vi "Main.vi"() -> ()   [LabVIEW 2019, in "GameEngine.lvlib"]
uses:
  GameEngine.lvlib
  Sprite/SpriteData.ctl
  VGA/data.ctl
  <vilib>/Platform/TimedLoop/XDataNode/timing_clust.ctl
  <vilib>/Platform/TimedLoop/XDataNode/nitl_modes.ctl
  <vilib>/Platform/TimedLoop/XDataNode/wakeup.ctl
  <vilib>/rvi/Emulation/niFpgaGetClockAttributes.vi
  <vilib>/rvi/Emulation/niFpgaSctlEmulationGetInTimedLoop.vi
  <vilib>/rvi/Emulation/niFpgaEmulationReportErrorSimple.vi
  <vilib>/rvi/interface/RandomDataEmulation/niFpgaRandomDataHandleErrors.vi
  <vilib>/rvi/Emulation/niFpgaProcessEmulError.vi
  <vilib>/rvi/Emulation/niFpgaCriticalErrorInLSC.vi
  <vilib>/rvi/eio/common/nirviEmuTemplateMethod_errors.vi
  <vilib>/rvi/Memory/Memory_Emulation/nirvimemoryFastEmulation.vi
  <vilib>/rvi/Memory/Memory_Emulation/nirvimemoryEmulation.vi
  <vilib>/rvi/Emulation/niFpgaEmulationIsFPGAContextNoSignature.vi
  <vilib>/rvi/DataTransferAndStorage/Container/Common/niFpgaContainerGetUniqueNameForEmu.vi
  <vilib>/rvi/errors/nirviReportUnexpectedCaseInternalError (U32).vi
  <vilib>/rvi/DataTransferAndStorage/Container/Common/niFpgaContainerExecOnDevCompGetState.vi
  <vilib>/rvi/Memory/Memory_Emulation/niFpgaMemoryEmulationCacheClearOnFirstRun.vi
  <vilib>/rvi/Memory/Memory_Emulation/nirvimemoryEmulationManagerCache_MakeExclusive.vi
  <vilib>/rvi/Memory/Memory_Emulation/niFpgaMemoryEmulationValidateCache.vi
  <vilib>/rvi/Memory/Memory_Emulation/nirvimemoryEmulationManagerCache_InsertValue.vi
  <vilib>/Utility/error.llb/Clear Errors.vi
  <vilib>/rvi/Memory/Memory_Emulation/nirvimemoryEmulationManagerCache_ReleaseExclusive.vi
  <vilib>/rvi/Memory/Memory_Emulation/nirvimemoryEmulationManagerCache_GetValue.vi
  <vilib>/rvi/Memory/Memory_Emulation/nirvimemoryEmulationManagerCache_SetValue.vi
  <vilib>/rvi/Emulation/niFpgaSctlEmulationResourceMgr.vi
  <vilib>/rvi/DataTransferAndStorage/Container/XNode/niFpgaContainer.xnode
  <vilib>/rvi/interface/RandomDataEmulation/nirviRandomDataFpgaReadWriteTemplate.vi
  <vilib>/eio/EIONode/EIONode.xnode
  <vilib>/platform/TimedLoop/XDataNode/XDataNode.xnode
  <vilib>/rvi/Memory/Memory_Emulation/niFpgaMemoryEmulationRefIn.vi
  <vilib>/Platform/TimedLoop/XDataNode/XDNodeRunTimeDep.lvlib
  Shared/Shared.lvlib
  Sprite/Sprite.lvlib
  VGA/VGA.lvlib
panel:
  in  "y_Shift":i16
  in  "x_Shift":i16
  out "SoundBufferTimeout":bool
  out "SoundBufferFlushing":bool
  in  "SoundBuffer_Flush":bool
  in  "Spritebuffer_ResetAddress":bool
  in  "FadeColor":fxp<+,3,3>
  in  "FadeRate":u32=308000
  in  "ColorShift":fxp<+,3,3>
  in  "Tilebuffer_ResetAddress":bool
  in  "Sprites":T1[](array[typedef])=[{"Pos_X"=0, "Pos_Y"=0, "Width"=0, "Height"=0, "BufferIndex"=0, "TransparencyColor"=0.0}, {"Pos_X"=0, "Pos_Y"=0, "Width"=0, "Height"=0, "BufferIndex"=0, "TransparencyColor"=0.0}, {"Pos_X"=0, "Pos_Y"=0, "Width"=0, "Height"=0, "BufferIndex"=0, "TransparencyColor"=0.0}]
  out "right_2":bool
  out "right_1":bool
  out "right_down":bool
  out "right_up":bool
  out "right_right":bool
  out "right_left":bool
  out "SystemButton":bool
  out "left_2":bool
  out "left_1":bool
  out "left_down":bool
  out "left_up":bool
  out "left_right":bool
  out "left_left":bool
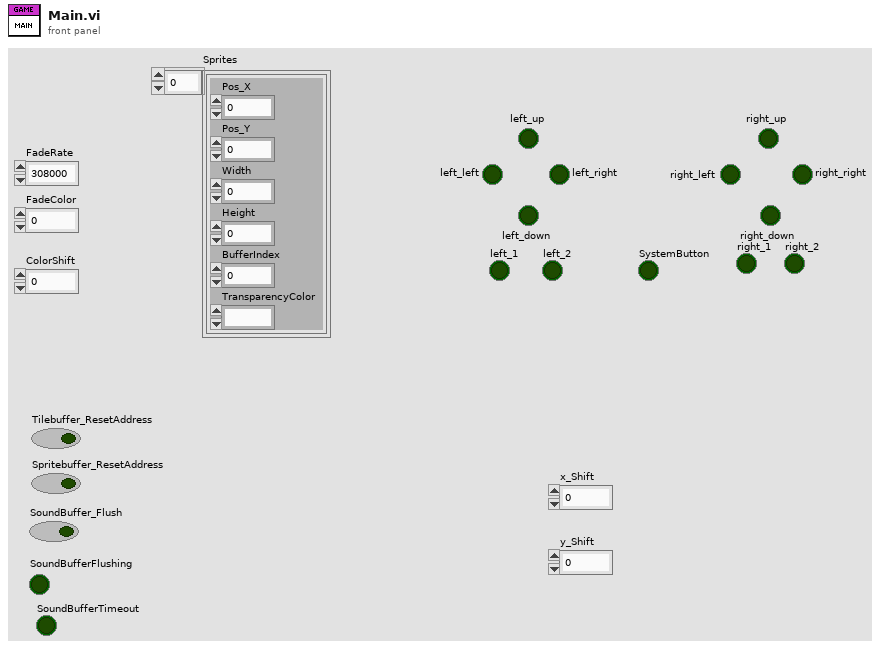
[diagram p1: front panel]
types:
  T1 = typedef "Sprite.lvlib/SpriteData.ctl" = cluster{"Pos_X":i16, "Pos_Y":i16, "Width":i16, "Height":i16, "BufferIndex":i16, "TransparencyColor":fxp<+,3,3>}
  T2 = typedef "VGA.lvlib/data.ctl" = cluster{"x_frontporch":u8, "x_syncpulse":u8, "x_backporch":u8, "y_frontporch":u8, "y_syncpulse":u8, "y_backporch":u8, "DrawPixel?":bool, "x_tickcount":u16, "y_tickcount":u16, "x_Index":i16, "y_Index":i16, "x_shift":i16}
  T3 = typedef "XDNodeRunTimeDep.lvlib/timing_clust.ctl" = cluster{"Expected End [f-1]":u64, "Actual End [f-1]":u64, "Finished Late? [f-1]":bool, "Expected End [i-1]":u64, "Actual End [i-1]":u64, "Finished Late? [i-1]":bool, "Expected Start [i]":u64, "Actual Start [i]":u64, "Expected Start [f]":u64, "Actual Start [f]":u64, "Source Name":string, "Structure Name":string, "Period":i64, "Deadline":i64, "Offset":i64, "Start":i64, "Priority":i32, "Timeout":i32, "Mode":T4, "Wakeup Reason":T5, "Error":errorcluster, "Source Type":string, "Secondary Source Type":string, "Global End Time":u64, "Global Start Time":u64, "Frame Duration":u64, "Iteration Duration":u64, "Assigned CPU":i32, "I/O Scan Engine Mode":u32}
  T4 = typedef "XDNodeRunTimeDep.lvlib/nitl_modes.ctl" = enum32{"No Change", "Process missed periods, maintain original phase", "Discard missed periods, maintain original phase", "Process missed periods, ignore original phase", "Discard missed periods, ignore original phase"}
  T5 = typedef "XDNodeRunTimeDep.lvlib/wakeup.ctl" = enum32{"Normal", "Aborted", "Asynchronous wakeup", "Timing source error", "Timed loop error", "Timeout"}
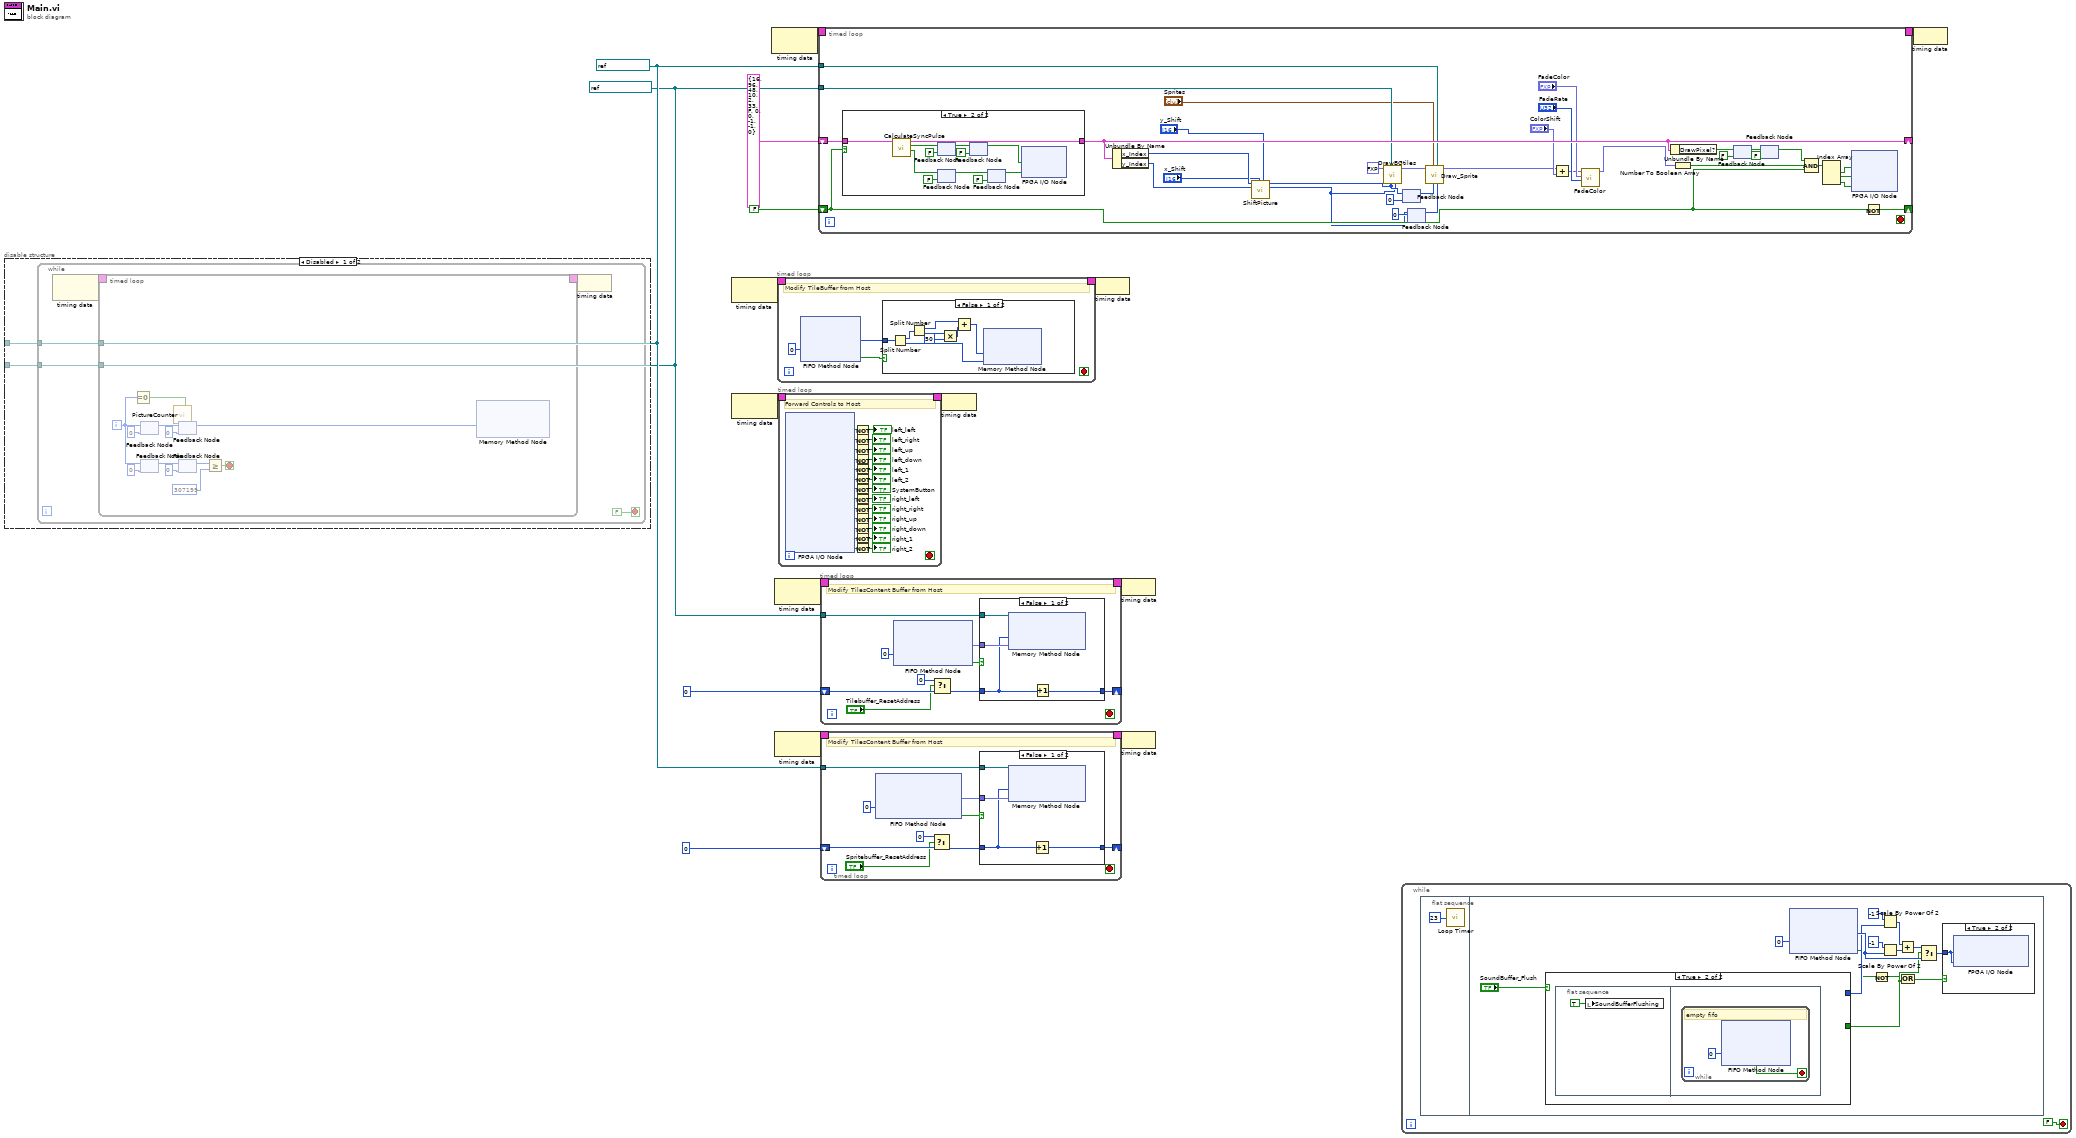
[diagram p0: block diagram]
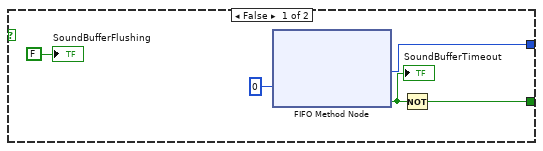
[diagram p8: hidden frame]
diagram:
  w2 = refnum<k21> "SpriteBuffer" ("SpriteBuffer")
  w1 = refnum<k21> "TileBufferLarge" ("Tilebuffer")
  n1 = disable-structure shown="Disabled" {
    disable-tunnel: w1 -> [w18 _]
    disable-tunnel: w2 -> [w17 _]
    frame Disabled {
      n2 = while {
        tunnel: w18 -> [w20]
        tunnel: w17 -> [w19]
        stop <- FALSE stop-if-true
        n3 = node-c288() -> (w23:T3)  [unwired: 1 in]
        n4 = timed-loop {
          timing: w23 -> [_]
          timing-out: [_] -> w22
          tunnel: w20 -> [w25]
          tunnel: w19 -> [w24]
          i -> [w29]
          stop <- w38 stop-if-true
          n5 = Equal To 0?(x=w29) -> (x = 0?=w26:bool)
          n6 = feedback #1(0) -> (w34:i32)
          n7 = feedback-in #1(w29) -> ()
          n8 = feedback #2(0) -> (w32:i32)
          n9 = feedback-in #2(w29) -> ()
          n10 = call "PictureCounter.vi"("Reset? (f)"=w26) -> ()  [unwired: 9 in, 2 out]
          n11 = feedback #3(0) -> (w28:i32)
          n12 = feedback-in #3(w34) -> ()
          n13 = feedback #4(0) -> (w35:i32)
          n14 = feedback-in #4(w32) -> ()
          n15 = Greater Or Equal?(x=w35, y=307199) -> (x >= y?=w38:bool)
          n16 = xnode ("Memory Method Node")("Address"=w28) -> ("Data"=w27:fxp<+,3,3>)  [unwired: 1 in, 1 out]
        }
        n17 = node-c288(w22) -> ()
      }
    }
    frame Enabled {
    }
  }
  n18 = node-c288() -> (w16:T3)  [unwired: 1 in]
  n19 = node-c288() -> (w14:T3)  [unwired: 1 in]
  n20 = node-c288() -> (w6:T3)  [unwired: 1 in]
  n21 = node-c288() -> (w12:T3)  [unwired: 1 in]
  n22 = node-c288() -> (w9:T3)  [unwired: 1 in]
  n23 = timed-loop {
    timing: w16 -> [_]
    timing-out: [_] -> w15
    stop <- _ stop-if-true
    # "Modify TileBuffer from Host"
    n24 = xnode ("FIFO Method Node")("Timeout"=0) -> ("Element"=w44:u64, "Timed Out?"=w43:bool)  [unwired: 1 in, 1 out]
    n25 = case shown="False" w43 {
      tunnel: w44 -> [w53 _]
      frame False {
        n26 = Split Number(x=w53) -> (hi(x)=w51:u32, lo(x)=w52:u32)
        n27 = Split Number(x=w51) -> (hi(x)=w47:u16, lo(x)=w50:u16)
        n28 = Multiply(x=w50, y=u8 50) -> (x*y=w48:u16)
        n29 = Add(x=w47, y=w48) -> (x+y=w46:u16)
        n30 = xnode ("Memory Method Node")("Address"=w46, "Data"=w52) -> ()  [unwired: 1 in, 1 out]
      }
      frame True {
      }
    }
  }
  n31 = timed-loop {
    timing: w14 -> [_]
    timing-out: [_] -> w13
    stop <- _ stop-if-true
    # "Forward Controls to Host"
    n32 = xnode "FPGA I/O Node"() -> ("left_left"=w81:bool, "left_right"=w80:bool, "left_up"=w79:bool, "left_down"=w78:bool, "left_1"=w77:bool, "left_2"=w76:bool, "SystemButton"=w75:bool, "right_left"=w74:bool, "right_right"=w73:bool, "right_up"=w72:bool, "right_down"=w71:bool, "right_1"=w70:bool, "right_2"=w69:bool)  [unwired: 13 in, 13 out]
    n33 = Not(x=w81) -> (.not. x?=→"left_left":bool)
    n34 = Not(x=w80) -> (.not. x?=→"left_right":bool)
    n35 = Not(x=w79) -> (.not. x?=→"left_up":bool)
    n36 = Not(x=w78) -> (.not. x?=→"left_down":bool)
    n37 = Not(x=w77) -> (.not. x?=→"left_1":bool)
    n38 = Not(x=w76) -> (.not. x?=→"left_2":bool)
    n39 = Not(x=w75) -> (.not. x?=→"SystemButton":bool)
    n40 = Not(x=w74) -> (.not. x?=→"right_left":bool)
    n41 = Not(x=w73) -> (.not. x?=→"right_right":bool)
    n42 = Not(x=w72) -> (.not. x?=→"right_up":bool)
    n43 = Not(x=w71) -> (.not. x?=→"right_down":bool)
    n44 = Not(x=w70) -> (.not. x?=→"right_1":bool)
    n45 = Not(x=w69) -> (.not. x?=→"right_2":bool)
  }
  n46 = timed-loop {
    timing: w6 -> [_]
    timing-out: [_] -> w5
    shift-right: [w113] -> _
    shift-left: T2 {"x_frontporch"=16, "x_syncpulse"=96, "x_backporch"=48, "y_frontporch"=10, "y_syncpulse"=2, "y_backporch"=33, "DrawPixel?"=FALSE, "x_tickcount"=0, "y_tickcount"=0, "x_Index"=-1, "y_Index"=-1, "x_shift"=0} ("VGA_data") -> [w118]
    shift-right: [w115] -> _
    shift-left: FALSE -> [w106]
    tunnel: w2 -> [w104]
    tunnel: w1 -> [w105]
    stop <- _ stop-if-true
    n47 = case shown="True" w106 {
      tunnel: w118 -> [w119 w131]
      tunnel: [w119 w130] -> w113
      frame False {
      }
      frame True {
        n48 = call "CalculateSyncPulse.vi"("VGA_data"=w131) -> ("vSync"=w129:bool, "hSync"=w128:bool, "VGA_data 2"=w130:T2)  [unwired: 8 in]
        n49 = feedback-in #5(w128) -> ()
        n50 = feedback #5(FALSE ("hSync")) -> (w127:bool)
        n51 = feedback-in #6(w129) -> ()
        n52 = feedback #6(FALSE ("vSync")) -> (w126:bool)
        n53 = feedback-in #7(w127) -> ()
        n54 = feedback #7(FALSE ("hSync")) -> (w122:bool)
        n55 = feedback-in #8(w126) -> ()
        n56 = feedback #8(FALSE ("vSync")) -> (w123:bool)
        n57 = xnode "FPGA I/O Node"("hSync"=w122, "vSync"=w123) -> ()  [unwired: 2 in, 2 out]
      }
    }
    n58 = Unbundle By Name(w113) -> ("x_Index"=w89:i16, "y_Index"=w88:i16)
    n59 = call "ShiftPicture.vi"("y_Shift"="y_Shift", "x_Shift"="x_Shift", "y_Index"=w88, "x_Index"=w89) -> ("y_index_shifted"=w86:i16, "x_index_shifted"=w87:i16)  [unwired: 6 in]
    n60 = call "DrawBGtiles.vi"("y"=w86, "x"=w87, "Tilebuffer"=w105, "color_in"=fxp<+,3,3> 0.0) -> ("color_out"=w93:fxp<+,3,3>)  [unwired: 7 in]
    n61 = feedback #9(i16 0 ("x_Index")) -> (w99:i16)
    n62 = feedback-in #9(w87) -> ()
    n63 = feedback #10(i16 0 ("y_Index")) -> (w100:i16)
    n64 = feedback-in #10(w86) -> ()
    n65 = call "Draw_Sprite.vi"("y_index"=w100, "SpriteBuffer"=w104, "x_index"=w99, "SpritesData"="Sprites", "color_in"=w93) -> ("color_out"=w94:fxp<+,3,3>)  [unwired: 6 in]
    n66 = Add(x=w94, y="ColorShift") -> (x+y=w95:fxp<+,3,3>)
    n67 = call "FadeColor.vi"("FadeRate"="FadeRate", "FadeColor in"="FadeColor", "Color in"=w95) -> ("FadeColor out"=w117:fxp<+,3,3>)  [unwired: 8 in]
    n68 = Unbundle By Name(w113) -> ("DrawPixel?"=w112:bool)
    n69 = Number To Boolean Array(number=w117) -> (Boolean array=w116:bool[])
    n70 = feedback #11(FALSE ("DrawPixel?")) -> (w108:bool)
    n71 = feedback-in #11(w112) -> ()
    n72 = feedback-in #12(w108) -> ()
    n73 = feedback #12(FALSE ("DrawPixel?")) -> (w103:bool)
    n74 = Compound Arithmetic op=AND(w103, w116, w106) -> (w114:bool[])
    n75 = Index Array(array=w114) -> (element #1=w111:bool, element #2=w110:bool, element #3=w109:bool)  [unwired: 3 in]
    n76 = xnode "FPGA I/O Node"("RED"=w111, "GREEN"=w110, "BLUE"=w109) -> ()  [unwired: 3 in, 3 out]
    n77 = Not(x=w106) -> (.not. x?=w115:bool)
  }
  n78 = timed-loop {
    timing: w12 -> [_]
    timing-out: [_] -> w11
    shift-right: [w138] -> _
    shift-left: u32 0 ("Address") -> [w139]
    tunnel: w1 -> [w134]
    stop <- _ stop-if-true
    # "Modify TilesContent Buffer from Host"
    n79 = xnode ("FIFO Method Node")("Timeout"=0) -> ("Element"=w140:fxp<+,3,3>, "Timed Out?"=w141:bool)  [unwired: 1 in, 1 out]
    n80 = Select(t=u32 0, s="Tilebuffer_ResetAddress", f=w139) -> (s? t:f=w137:u32)
    n81 = case shown="False" w141 {
      tunnel: w140 -> [w146 _]
      tunnel: [w145 w147] -> w138
      tunnel: w137 -> [w144 w147]
      tunnel: w134 -> [w143 _]
      frame False {
        n82 = xnode ("Memory Method Node")("Address"=w144, "Data"=w146, "Memory In"=w143) -> ()  [unwired: 1 out]
        n83 = Increment(x=w144) -> (x+1=w145:u32)
      }
      frame True {
      }
    }
  }
  n84 = timed-loop {
    timing: w9 -> [_]
    timing-out: [_] -> w8
    shift-right: [w154] -> _
    shift-left: u32 0 ("Address") -> [w155]
    tunnel: w2 -> [w150]
    stop <- _ stop-if-true
    # "Modify TilesContent Buffer from Host"
    n85 = xnode ("FIFO Method Node")("Timeout"=0) -> ("Element"=w156:fxp<+,3,3>, "Timed Out?"=w157:bool)  [unwired: 1 in, 1 out]
    n86 = Select(t=u32 0, s="Spritebuffer_ResetAddress", f=w155) -> (s? t:f=w153:u32)
    n87 = case shown="False" w157 {
      tunnel: w156 -> [w162 _]
      tunnel: [w161 w163] -> w154
      tunnel: w153 -> [w160 w163]
      tunnel: w150 -> [w159 _]
      frame False {
        n88 = xnode ("Memory Method Node")("Address"=w160, "Data"=w162, "Memory In"=w159) -> ()  [unwired: 1 out]
        n89 = Increment(x=w160) -> (x+1=w161:u32)
      }
      frame True {
      }
    }
  }
  n90 = node-c288(w13) -> ()
  n91 = node-c288(w15) -> ()
  n92 = node-c288(w11) -> ()
  n93 = node-c288(w8) -> ()
  n94 = while {
    stop <- FALSE stop-if-true
    n95 = flat-sequence {
      frame #0 {
        n96 = call "Loop Timer"("Count(uSec)"=u32 23) -> ()  [unwired: 1 out]
      }
      frame #1 {
        n97 = case shown="True" "SoundBuffer_Flush" {
          tunnel: [w183 _] -> w171
          tunnel: [w184 _] -> w177
          frame False {
            n98 = xnode ("FIFO Method Node")("Timeout"=0) -> ("Element"=w184:i16, "Timed Out?"=w185:bool)  [unwired: 1 in, 1 out]
            "SoundBufferTimeout" <- w185
            n99 = Not(x=w185) -> (.not. x?=w183:bool)
            "SoundBufferFlushing" <- FALSE ("SoundBufferFlushing")
          }
          frame True {
            n100 = flat-sequence {
              frame #0 {
                n101 = local write "SoundBufferFlushing"(TRUE ("SoundBufferFlushing")) -> ()
              }
              frame #1 {
                n102 = while {
                  stop <- w190 stop-if-true
                  # "empty fifo"
                  n103 = xnode ("FIFO Method Node")("Timeout"=0) -> ("Timed Out?"=w190:bool)  [unwired: 1 in, 2 out]
                }
              }
            }
          }
        }
        n104 = xnode ("FIFO Method Node")("Timeout"=0) -> ("Element"=w178:i16, "Timed Out?"=w169:bool)  [unwired: 1 in, 1 out]
        n105 = Not(x=w169) -> (.not. x?=w168:bool)
        n106 = Scale By Power Of 2(n=i16 -1, x=w177) -> (x*2^n=w173:i16)
        n107 = Scale By Power Of 2(n=i16 -1, x=w178) -> (x*2^n=w174:i16)
        n108 = Add(x=w173, y=w174) -> (x+y=w172:i16)
        n109 = Or(x=w168, y=w171) -> (x .or. y?=w170:bool)
        n110 = Select(t=w172, s=w171, f=w178) -> (s? t:f=w179:i16)
        n111 = case shown="True" w170 {
          tunnel: w179 -> [_ w182]
          frame False {
          }
          frame True {
            n112 = xnode "FPGA I/O Node"("AudioOut/Left"=w182, "AudioOut/Right"=w182) -> ()  [unwired: 2 in, 2 out]
          }
        }
      }
    }
  }
  n113 = node-c288(w5) -> ()
